vi "test_libssh2_sftp_fstatvfs.vi"() -> ()   [LabVIEW 2017, in "integration_tests.lvlib"]
uses:
  integration_tests.lvlib
  support/support.lvlib
  libssh2/libssh2.lvlib
  <vilib>/PNR/Transparent Assertions/Transparent Assertions/Transparent Assertions.lvlib
panel:
  out "error out":errorcluster
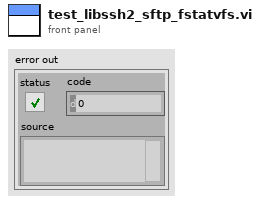
[diagram p1: front panel]
types:
  T1 = typedef "libssh2.lvlib/Session Refnum.ctl" = refnum<k1>
  T2 = typedef "libssh2.lvlib/SFTP Refnum.ctl" = refnum<k1>
  T3 = typedef "libssh2.lvlib/SFTP Handle Refnum.ctl" = refnum<k1>
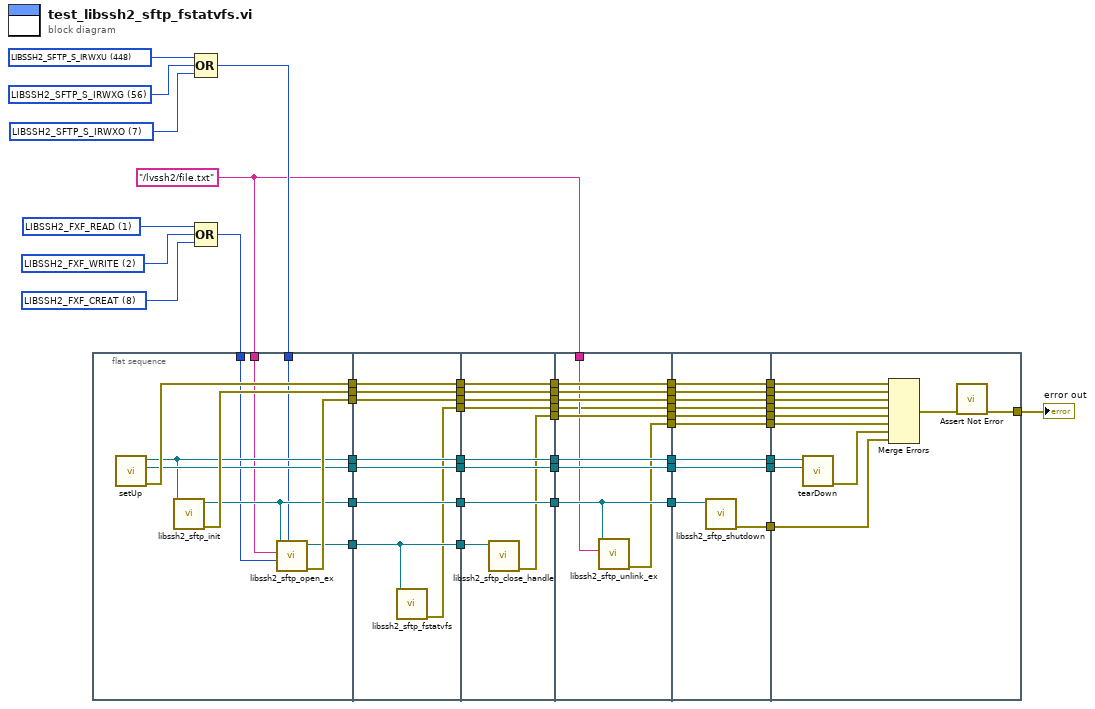
[diagram p0: block diagram]
diagram:
  w47 = u32 2 items=["LIBSSH2_FXF_READ"=1, "LIBSSH2_FXF_WRITE"=2, "LIBSSH2_FXF_APPEND"=4, "LIBSSH2_FXF_CREAT"=8, "LIBSSH2_FXF_TRUNC"=16, "LIBSSH2_FXF_EXCL"=32] ("flags")
  w48 = u32 1 items=["LIBSSH2_FXF_READ"=1, "LIBSSH2_FXF_WRITE"=2, "LIBSSH2_FXF_APPEND"=4, "LIBSSH2_FXF_CREAT"=8, "LIBSSH2_FXF_TRUNC"=16, "LIBSSH2_FXF_EXCL"=32] ("flags")
  w46 = u32 8 items=["LIBSSH2_FXF_READ"=1, "LIBSSH2_FXF_WRITE"=2, "LIBSSH2_FXF_APPEND"=4, "LIBSSH2_FXF_CREAT"=8, "LIBSSH2_FXF_TRUNC"=16, "LIBSSH2_FXF_EXCL"=32] ("flags")
  w5 = "/lvssh2/file.txt" ("filename")
  w49 = 7 items=["LIBSSH2_SFTP_S_IRWXU"=448, "LIBSSH2_SFTP_S_IRUSR"=256, "LIBSSH2_SFTP_S_IWUSR"=128, "LIBSSH2_SFTP_S_IXUSR"=64, "LIBSSH2_SFTP_S_IRWXG"=56, "LIBSSH2_SFTP_S_IRGRP"=32, "LIBSSH2_SFTP_S_IWGRP"=16, "LIBSSH2_SFTP_S_IXGRP"=8, "LIBSSH2_SFTP_S_IRWXO"=7, "LIBSSH2_SFTP_S_IROTH"=4, "LIBSSH2_SFTP_S_IWOTH"=2, "LIBSSH2_SFTP_S_IXOTH"=1] ("mode")
  w50 = 56 items=["LIBSSH2_SFTP_S_IRWXU"=448, "LIBSSH2_SFTP_S_IRUSR"=256, "LIBSSH2_SFTP_S_IWUSR"=128, "LIBSSH2_SFTP_S_IXUSR"=64, "LIBSSH2_SFTP_S_IRWXG"=56, "LIBSSH2_SFTP_S_IRGRP"=32, "LIBSSH2_SFTP_S_IWGRP"=16, "LIBSSH2_SFTP_S_IXGRP"=8, "LIBSSH2_SFTP_S_IRWXO"=7, "LIBSSH2_SFTP_S_IROTH"=4, "LIBSSH2_SFTP_S_IWOTH"=2, "LIBSSH2_SFTP_S_IXOTH"=1] ("mode")
  w51 = 448 items=["LIBSSH2_SFTP_S_IRWXU"=448, "LIBSSH2_SFTP_S_IRUSR"=256, "LIBSSH2_SFTP_S_IWUSR"=128, "LIBSSH2_SFTP_S_IXUSR"=64, "LIBSSH2_SFTP_S_IRWXG"=56, "LIBSSH2_SFTP_S_IRGRP"=32, "LIBSSH2_SFTP_S_IWGRP"=16, "LIBSSH2_SFTP_S_IXGRP"=8, "LIBSSH2_SFTP_S_IRWXO"=7, "LIBSSH2_SFTP_S_IROTH"=4, "LIBSSH2_SFTP_S_IWOTH"=2, "LIBSSH2_SFTP_S_IXOTH"=1] ("mode")
  n1 = flat-sequence {
    tunnel: [w61] -> w38
    tunnel: [w60] -> w37
    tunnel: [w59] -> w36
    tunnel: [w58] -> w35
    tunnel: [w57] -> w34
    tunnel: [w56] -> w33
    tunnel: [w52] -> w32
    tunnel: w24 -> [w53]
    tunnel: w5 -> [w54]
    tunnel: w23 -> [w55]
    tunnel: w38 -> [w69]
    tunnel: [w69] -> w31
    tunnel: w37 -> [w68]
    tunnel: [w68] -> w30
    tunnel: w36 -> [w67]
    tunnel: [w67] -> w29
    tunnel: w35 -> [w66]
    tunnel: [w66] -> w28
    tunnel: w34 -> [w65]
    tunnel: [w65] -> w27
    tunnel: w33 -> [w64]
    tunnel: [w64] -> w26
    tunnel: w32 -> [w63]
    tunnel: [w63] -> w25
    tunnel: [w62] -> w4
    tunnel: [w72] -> w9
    tunnel: w31 -> [w78]
    tunnel: [w78] -> w11
    tunnel: w30 -> [w77]
    tunnel: [w77] -> w13
    tunnel: w29 -> [w76]
    tunnel: [w76] -> w15
    tunnel: w28 -> [w75]
    tunnel: [w75] -> w17
    tunnel: w27 -> [w74]
    tunnel: [w74] -> w19
    tunnel: w26 -> [w73]
    tunnel: [w73] -> w21
    tunnel: w25 -> [w71]
    tunnel: w4 -> [w70]
    tunnel: [w70] -> w3
    tunnel: w21 -> [w88]
    tunnel: [w88] -> w20
    tunnel: w19 -> [w87]
    tunnel: [w87] -> w18
    tunnel: w17 -> [w82]
    tunnel: [w82] -> w16
    tunnel: w15 -> [w86]
    tunnel: [w86] -> w14
    tunnel: w13 -> [w85]
    tunnel: [w85] -> w12
    tunnel: w11 -> [w84]
    tunnel: [w84] -> w10
    tunnel: w9 -> [w83]
    tunnel: [w83] -> w8
    tunnel: [w81] -> w7
    tunnel: w5 -> [w80]
    tunnel: w3 -> [w79]
    tunnel: [w79] -> w2
    tunnel: w20 -> [w98]
    tunnel: [w98] -> w45
    tunnel: w18 -> [w97]
    tunnel: [w97] -> w44
    tunnel: w16 -> [w94]
    tunnel: w14 -> [w96]
    tunnel: [w96] -> w43
    tunnel: w12 -> [w95]
    tunnel: [w95] -> w42
    tunnel: [w93] -> w41
    tunnel: w10 -> [w92]
    tunnel: [w92] -> w40
    tunnel: [w91] -> w39
    tunnel: w8 -> [w91]
    tunnel: w7 -> [w90]
    tunnel: [w90] -> w6
    tunnel: w2 -> [w89]
    tunnel: [w89] -> w1
    tunnel: w45 -> [w110]
    tunnel: w44 -> [w109]
    tunnel: w43 -> [w108]
    tunnel: w42 -> [w105]
    tunnel: w41 -> [w104]
    tunnel: w40 -> [w103]
    tunnel: w39 -> [w102]
    tunnel: [w101] -> w22
    tunnel: w6 -> [w100]
    tunnel: w1 -> [w99]
    frame #0 {
      n2 = call "setUp.vi"() -> ("error out"=w59:errorcluster, "connection ID"=w57:refnum<k5>, "session"=w56:T1)  [unwired: 9 in]
      n3 = call "libssh2_sftp_init.vi"("session"=w56) -> ("error out"=w60:errorcluster, "sftp"=w58:T2)  [unwired: 9 in]
      n4 = call "libssh2_sftp_open_ex.vi"("mode"=w55, "flags"=w53, "filename"=w54, "sftp"=w58) -> ("error out"=w61:errorcluster, "sftp handle"=w52:T3)  [unwired: 6 in]
    }
    frame #1 {
      n5 = call "libssh2_sftp_fstatvfs.vi"("sftp handle"=w63) -> ("error out"=w62:errorcluster)  [unwired: 9 in, 1 out]
    }
    frame #2 {
      n6 = call "libssh2_sftp_close_handle.vi"("sftp handle"=w71) -> ("error out"=w72:errorcluster)  [unwired: 10 in]
    }
    frame #3 {
      n7 = call "libssh2_sftp_unlink_ex.vi"("file"=w80, "sftp"=w82) -> ("error out"=w81:errorcluster)  [unwired: 9 in]
    }
    frame #4 {
      n8 = call "libssh2_sftp_shutdown.vi"("sftp"=w94) -> ("error out"=w93:errorcluster)  [unwired: 10 in]
    }
    frame #5 {
      n9 = call "tearDown.vi"("connection ID"=w109, "session"=w110) -> ("error out"=w107:errorcluster)  [unwired: 9 in]
      n10 = Merge Errors(w108, w105, w103, w99, w102, w100, w107, w104) -> (w106:errorcluster)
      n11 = call <vilib>:"Assert Not Error.vi"("error in (no error)"=w106) -> ("error out"=w101:errorcluster)  [unwired: 10 in]
    }
  }
  n12 = Compound Arithmetic op=OR(w51, w50, w49) -> (w23:i32)
  n13 = Compound Arithmetic op=OR(w48, w47, w46) -> (w24:u32)
  "error out" <- w22
